vi "Shutdown Camera.vi"(8 "error in (no error)":errorcluster, 11 "CCDCamera in":refnum<class "CCDCamera.lvclass">) -> (0 "error out":errorcluster, 3 "CCDCamera out":refnum<class "CCDCamera.lvclass">)   [LabVIEW 2018, in "CCDCamera.lvclass"]
uses:
  CCDCamera.lvclass
  <userlib>/atmcd32d.llb/Shutter_type typedef.ctl
  <userlib>/atmcd32d.llb/Shutter_mode typedef.ctl
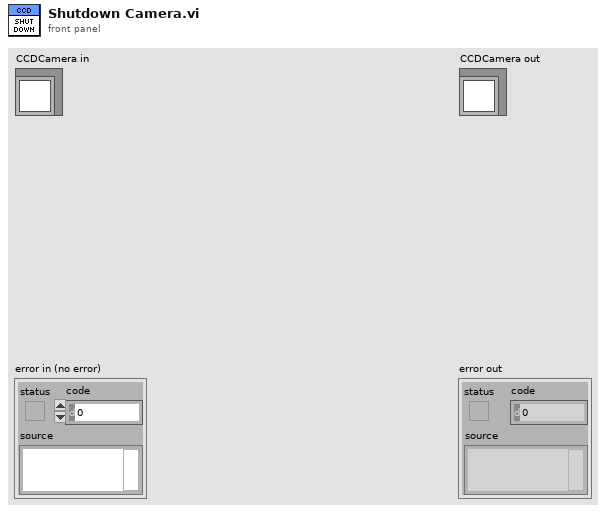
[diagram p1: front panel]
types:
  T1 = typedef "Shutter_mode typedef.ctl" = enum16{"Auto", "Open", "Close", "N/A (3)", "Open FVB Series", "Open Any Series"}
  T2 = typedef "Shutter_type typedef.ctl" = enum16{"TTL Low", "TTL High"}
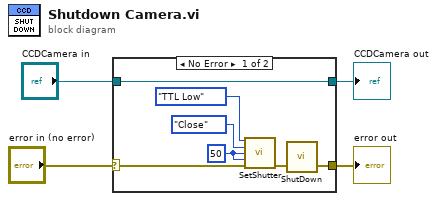
[diagram p0: block diagram]
diagram:
  n1 = case shown="No Error" "error in (no error)" {
    selector: "error in (no error)" -> [w10 w13]
    tunnel: [w8 w13] -> w3
    tunnel: [w11 w12] -> w1
    tunnel: "CCDCamera in" -> [w11 w12]
    frame No Error {
      w5 = 50 ("closingtime")
      n2 = call <userlib>:"SetShutter.vi"("type"=Shutter_type_typedef."TTL Low", "mode"=Shutter_mode_typedef."Close", "closingtime"=w5, "openingtime"=w5, "error in (no error)"=w10) -> ("error out"=w9:errorcluster)  [unwired: 9 in, 1 out]
      n3 = call <userlib>:"ShutDown.vi"("error in (no error)"=w9) -> ("error out"=w8:errorcluster)  [unwired: 1 in, 1 out]
    }
    frame Error {
    }
  }
  "error out" <- w3
  "CCDCamera out" <- w1
